vi "Uim Grob Reg wrapper.vi"(8 "error in (no error)":errorcluster caption="错误输入（无错误）", 9 "iLen":i32=1024, 11 "dwDevIndex":u32) -> (0 "error out":errorcluster caption="错误输出", 2 "pCanNodeIdList out":u32[](array[numeric]), 3 "function return":u32)   [LabVIEW 2016, in "UISimCanFunc_wrapper.lvlib"]
doc: "_declspec (dllexport) DWORD UimGrobReg_wrapper(DWORD dwDevIndex, DWORD pCanNodeIdList[], int iLen);"
uses:
  <userlib>/UISimCanFunc_wrapper/UISimCanFunc_wrapper.lvlib
  <userlib>/UISimCanFunc_wrapper/UISimCanFunc_wrapper.dll
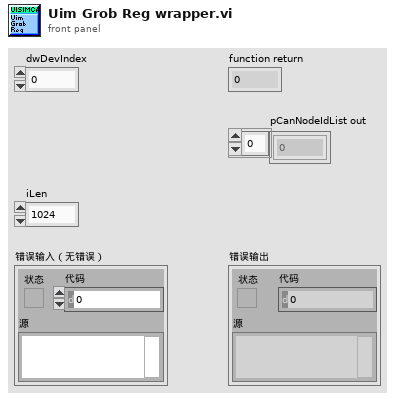
[diagram p1: front panel]
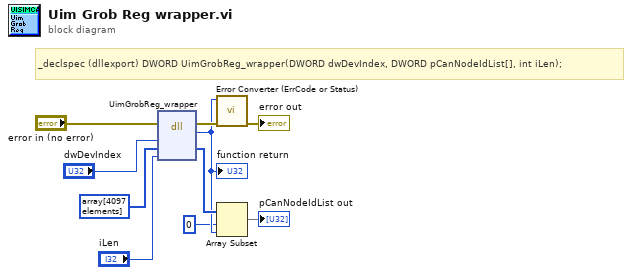
[diagram p0: block diagram]
diagram:
  # "_declspec (dllexport) DWORD UimGrobReg_wrapper(DWORD dwDevIndex, DWORD pCanNodeIdList[], int iLen);"
  n1 = dll-call lib="C:/Program Files (x86)/National Instruments/LabVIEW 2016/user.lib/UISimCanFunc_wrapper/UISimCanFunc_wrapper.*" fn="UimGrobReg_wrapper"(error in="error in (no error)", "dwDevIndex"="dwDevIndex", "pCanNodeIdList"=u32[] array[4097 elements], "iLen"="iLen") -> (error out=w6:errorcluster, w3:u32, "pCanNodeIdList"=w4:u32[])  [unwired: 4 in, 1 out]
  "function return" <- w3
  n2 = call <userlib>:"Error Converter (ErrCode or Status).vi"("error in (no error)"=w6, "error code"=w3) -> ("error out"=→"error out":errorcluster)  [unwired: 9 in]
  n3 = Array Subset(array=w4, index=0 ("索引"), length=w3) -> (→"pCanNodeIdList out":u32[])
